vi "AC Test Host.vi"() -> ()   [LabVIEW 2012]
uses:
  <vilib>/FPGAPlugInAG/PCI-7831R/niLvFpga_Open_PCI-7831R.vi
  <vilib>/rvi/interface/common/dynamic/niFpgaDynamicAddResources.vi
  <vilib>/Utility/error.llb/Error Cluster From Error Code.vi
  <vilib>/rvi/errors/niLvFpgaAdjustHostInterfaceError.vi
  <vilib>/FPGAPlugInAG/Dynamic/niLvFpga_Abort_Dynamic.vi
  <vilib>/FPGAPlugInAG/Dynamic/niLvFpga_Close_Dynamic.vi
  <vilib>/rvi/interface/nirviOpenFPGA/nirviOpenFPGA.xnode
  FPGA Bitfiles/Apporach-Retract_FPGATarget_InputOutputACSig_WF5RXjnepiw.lvbitx
  <vilib>/rvi/interface/nirviReadWriteControl/nirviReadWriteControl.xnode
  <vilib>/rvi/interface/nirviMethod/nirviMethod.xnode
  <vilib>/rvi/interface/nirviCloseFPGA/nirviCloseFPGA.xnode
  NiFpgaLv.dll
  <vilib>/rvi/interface/Simulation/niFpgaSimulationCallBeginRW.vi
panel:
  out "Numeric":dbl
  out "Input":dbl(graph)
  out "Output":dbl(graph)
  in  "Phase Shift":dbl
  in  "Frequency":i32
  in  "Stop":bool
  out "Converted Voltage":dbl
  in  "Sine Voltage":dbl
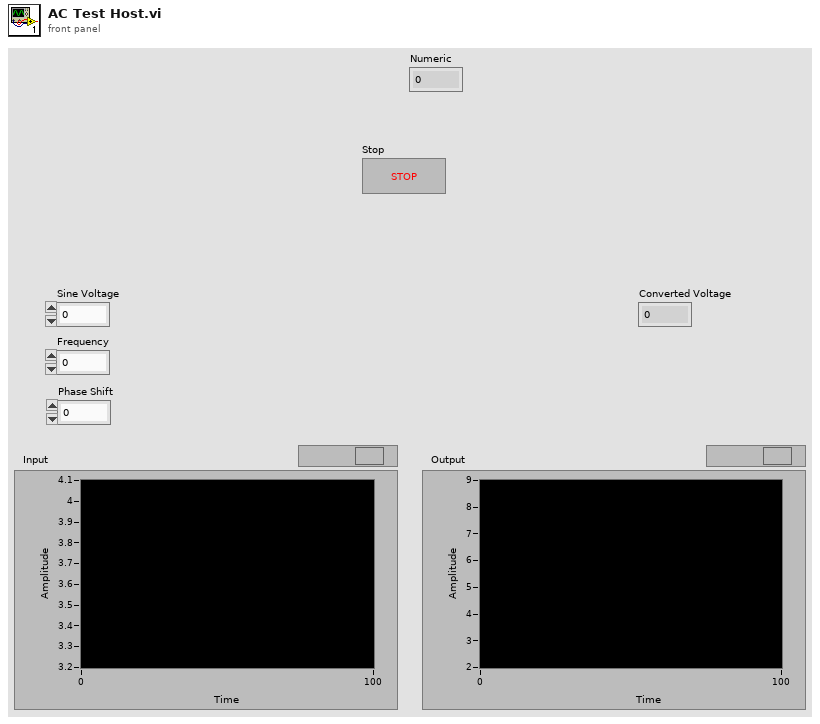
[diagram p1: front panel]
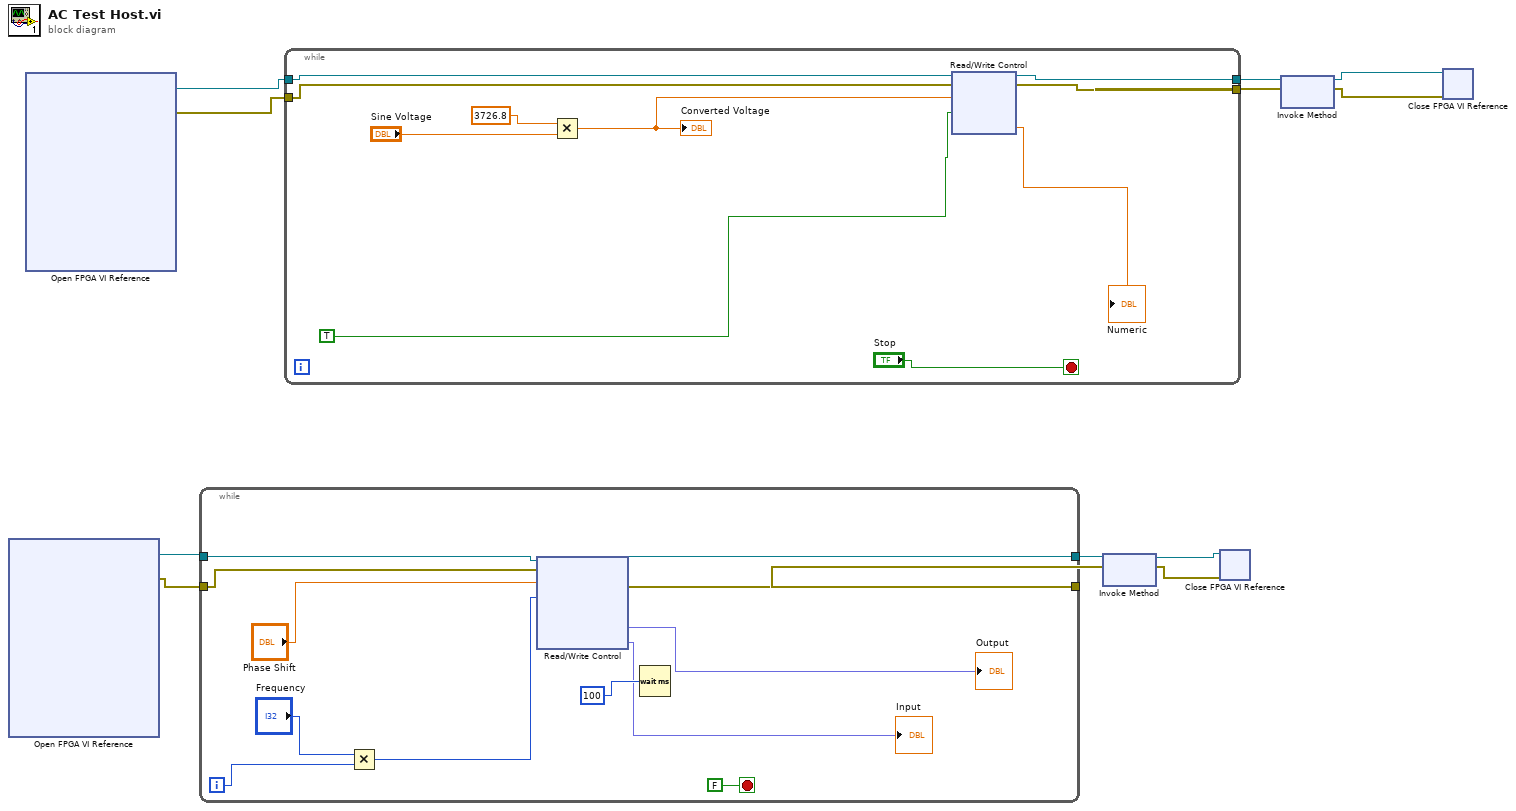
[diagram p0: block diagram]
diagram:
  n1 = xnode "Open FPGA VI Reference"() -> ("FPGA VI Reference Out"=w6:refnum<k20>, "error out"=w5:errorcluster)  [unwired: 2 in]
  n2 = xnode "Open FPGA VI Reference"() -> ("FPGA VI Reference Out"=w12:refnum<k20>, "error out"=w11:errorcluster)  [unwired: 2 in]
  n3 = while {
    tunnel: w6 -> [w22]
    tunnel: w5 -> [w21]
    tunnel: [w20] -> w4
    tunnel: [w19] -> w3
    i -> [w24]
    stop <- FALSE stop-if-true
    n4 = Multiply(x="Frequency", y=w24) -> (x*y=w18:i32)
    n5 = xnode "Read/Write Control"("FPGA VI Reference In"=w22, "error in"=w21, "Phase Shift"="Phase Shift", "Frequency"=w18) -> ("FPGA VI Reference Out"=w20:refnum<k20>, "error out"=w19:errorcluster, "Output Signal"=→"Output":fxp<+/-,26,16>, "Input Signal"=→"Input":fxp<+/-,26,16>)  [unwired: 1 in]
    n6 = Wait (ms)(milliseconds to wait=100) -> ()  [unwired: 1 out]
  }
  n7 = while {
    tunnel: w12 -> [w34]
    tunnel: w11 -> [w33]
    tunnel: [w32] -> w10
    tunnel: [w31] -> w9
    stop <- "Stop" stop-if-true
    n8 = Multiply(x=3726.8, y="Sine Voltage") -> (x*y=w27:dbl)
    "Converted Voltage" <- w27
    n9 = xnode "Read/Write Control"("FPGA VI Reference In"=w34, "error in"=w33, "Voltage"=w27, "Start"=TRUE ("Start Target")) -> ("FPGA VI Reference Out"=w32:refnum<k20>, "error out"=w31:errorcluster, "Numeric"=→"Numeric":sgl)
  }
  n10 = xnode "Invoke Method"("FPGA VI Reference In"=w4, "error in"=w3) -> ("FPGA VI Reference Out"=w2:refnum<k20>, "error out"=w1:errorcluster)
  n11 = xnode "Close FPGA VI Reference"("FPGA VI Reference In"=w2, "error in"=w1) -> ()  [unwired: 1 out]
  n12 = xnode "Invoke Method"("FPGA VI Reference In"=w10, "error in"=w9) -> ("FPGA VI Reference Out"=w8:refnum<k20>, "error out"=w7:errorcluster)
  n13 = xnode "Close FPGA VI Reference"("FPGA VI Reference In"=w8, "error in"=w7) -> ()  [unwired: 1 out]
